vi "Constraint_MinMax_New.vi"() -> (3 "TRAJ_CONSTAINT_MIN_MAX":T1)   [LabVIEW 2019, in "Trajectory_Library.lvlib"]
doc: "Constructs a MinMax with default values."
uses:
  Trajectory_Library.lvlib
  TRAJ_CONSTRAINT_MINMAX.ctl
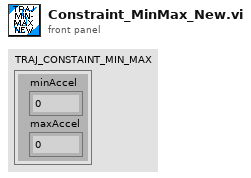
[diagram p1: front panel]
types:
  T1 = typedef "Trajectory_Library.lvlib/TRAJ_CONSTRAINT_MINMAX.ctl" = cluster{"minAccel":dbl, "maxAccel":dbl}
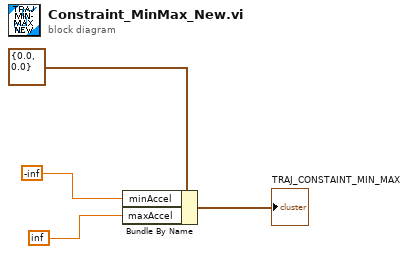
[diagram p0: block diagram]
diagram:
  n1 = Bundle By Name(cluster=T1 {"minAccel"=0.0, "maxAccel"=0.0} ("TRAJ_CONSTAINT_MIN_MAX"), "minAccel"=-inf, "maxAccel"=inf) -> (→"TRAJ_CONSTAINT_MIN_MAX":T1)
